vi "get_wavelengths.vi"(9 "wl end":dbl, 10 "wl start":dbl, 11 "file path (dialog if empty)":path) -> (2 "Wavelengths":dbl[](array[numeric]), 5 "length":dbl, 7 "start":dbl)   [LabVIEW 2019]
uses:
  <vilib>/Utility/file.llb/Read Delimited Spreadsheet (DBL).vi
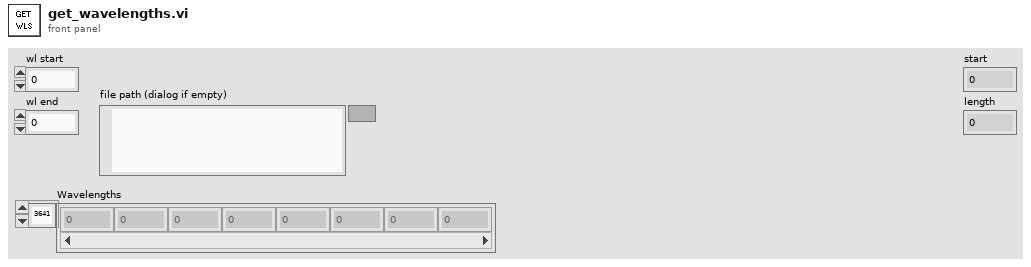
[diagram p1: front panel]
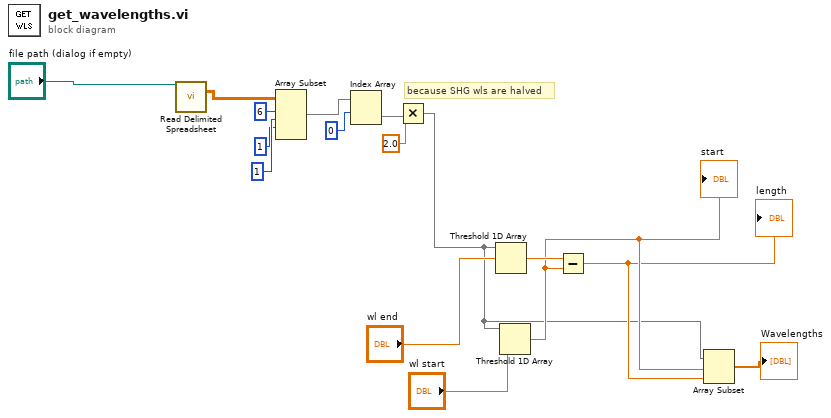
[diagram p0: block diagram]
diagram:
  # "because SHG wls are halved"
  n1 = call-poly <vilib>:"Read Delimited Spreadsheet.vi"("file path (dialog if empty)"="file path (dialog if empty)") -> ("all rows"=w16:dbl[][])  [unwired: 9 in, 5 out]
  n2 = Array Subset(array=w16, index (row)=6 ("index"), length (row)=1 ("length"), index (col)=1 ("index")) -> (w12:dbl[][])  [unwired: 1 in]
  n3 = Index Array(array=w12, index (row)=0) -> (element=w2:dbl[])  [unwired: 1 in]
  n4 = Multiply(x=w2, y=2.0) -> (x*y=w1:dbl[])
  n5 = Threshold 1D Array(2:"wl end", 3:w1) -> (0:w7:dbl)  [unwired: 1 in]
  n6 = Threshold 1D Array(2:"wl start", 3:w1) -> (0:w6:dbl)  [unwired: 1 in]
  "start" <- w6
  n7 = Subtract(x=w7, y=w6) -> (x-y=w5:dbl)
  "length" <- w5
  n8 = Array Subset(array=w1, index=w6, length=w5) -> (→"Wavelengths":dbl[])
